vi "SDF Alarms.vi"(0 "Str Refnum":refnum<vi>, 5 "DigNum Refnum":refnum<vi>, 7 "High High":dbl, 9 "High":dbl, 11 "LC-test":dbl, 12 "LOW":dbl, 13 "LOW LOW":dbl, 14 "Reset":bool) -> (4 "String":string, 6 "Alarm":bool, 8 "Alarm Horn":bool, 10 "Warning Horn":bool, 15 "Warning":bool)   [LabVIEW 2013]
panel:
  out "Alarm Lolo":bool
  out "Alarm Hihi":bool
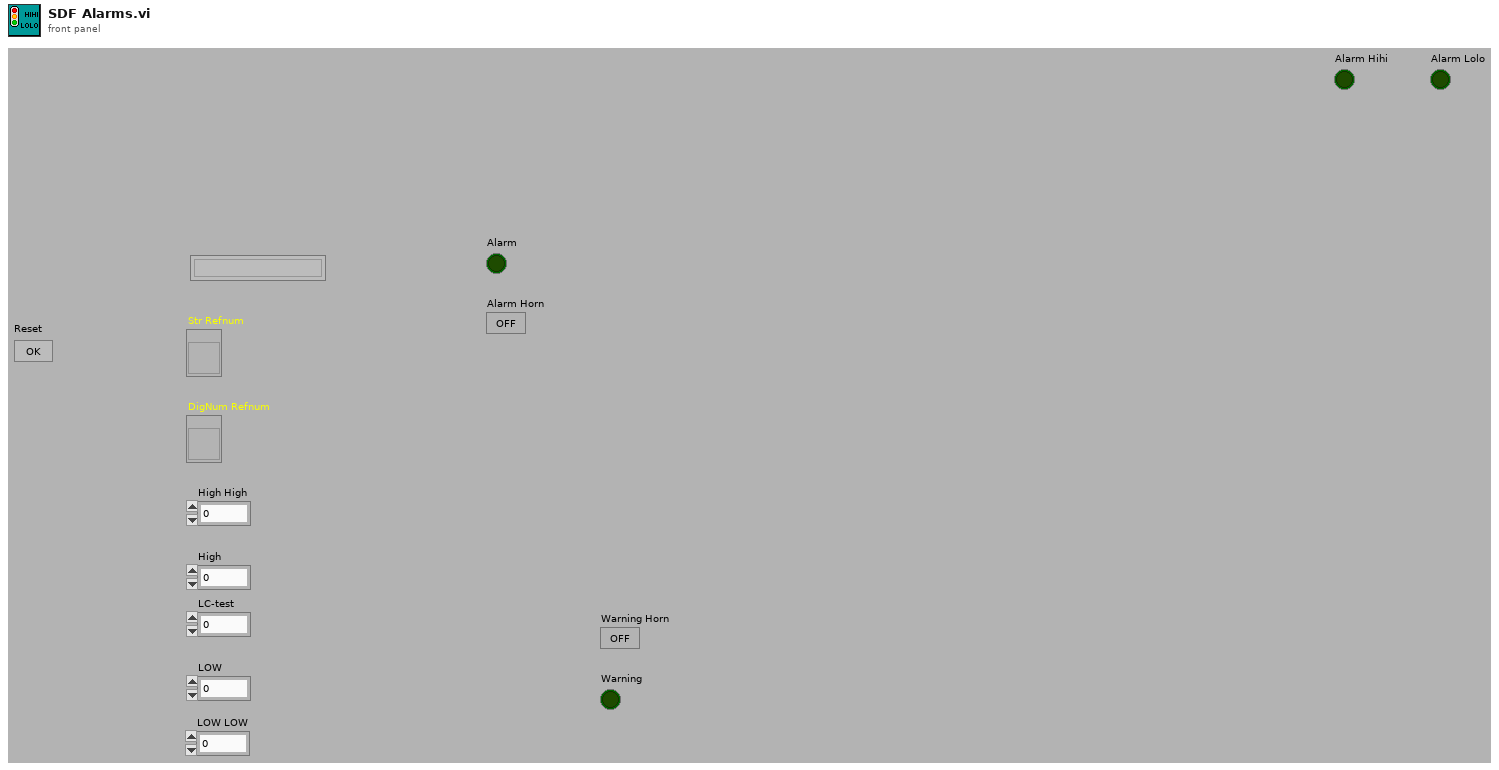
[diagram p1: front panel]
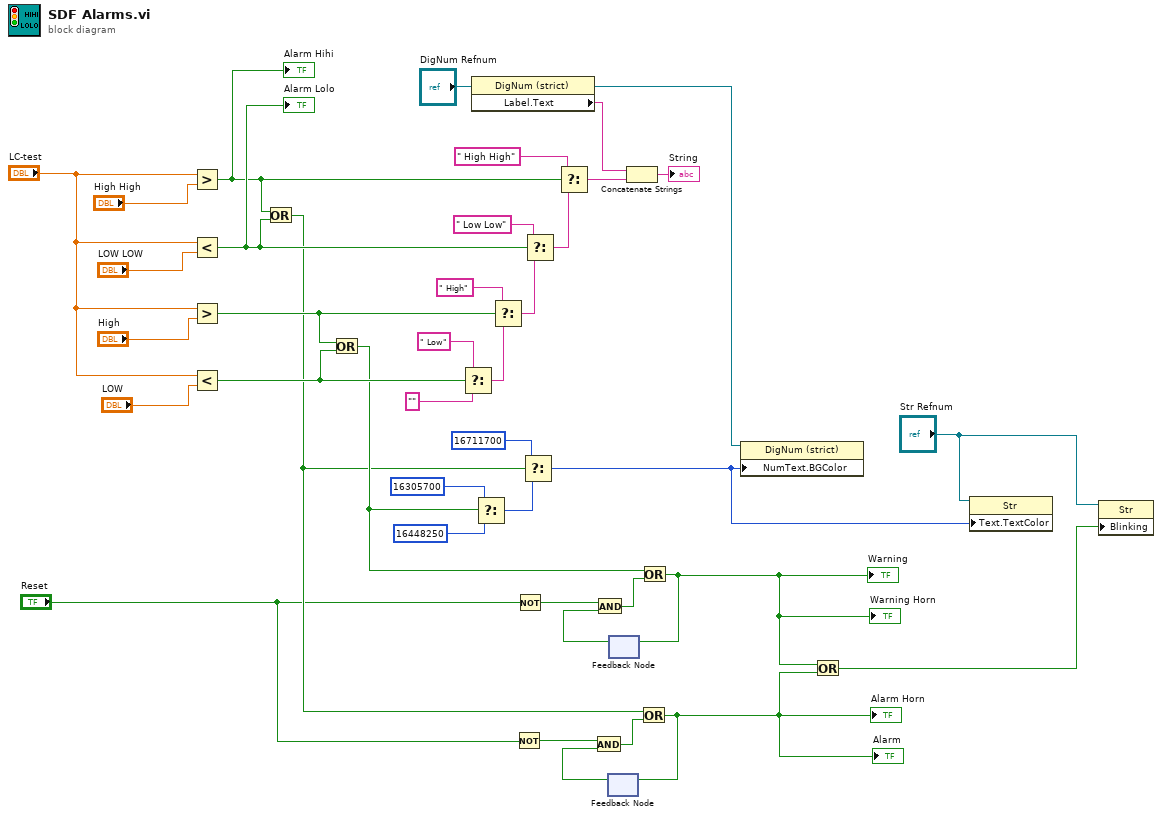
[diagram p0: block diagram]
diagram:
  n1 = Greater?(x="LC-test", y="High High") -> (0:w20:bool)
  "Alarm Hihi" <- w20
  n2 = Less?(x="LC-test", y="LOW LOW") -> (x < y?=w21:bool)
  "Alarm Lolo" <- w21
  n3 = Greater?(x="LC-test", y="High") -> (0:w28:bool)
  n4 = Less?(x="LC-test", y="LOW") -> (x < y?=w37:bool)
  n5 = Or(x=w20, y=w21) -> (x .or. y?=w9:bool)
  n6 = Or(x=w28, y=w37) -> (x .or. y?=w10:bool)
  n7 = Select(t=" Low", s=w37, f="") -> (s? t:f=w29:string)
  n8 = property on="Property Node" class="DigNum (strict)"(reference="DigNum Refnum") -> ("Label.Text"=w4:string)  [unwired: 1 in, 2 out]
  n9 = Select(t=16305700, s=w10, f=16448250) -> (s? t:f=w12:i32)
  n10 = Select(t=" High", s=w28, f=w29) -> (s? t:f=w30:string)
  n11 = Not(x="Reset") -> (.not. x?=w23:bool)
  n12 = Not(x="Reset") -> (.not. x?=w26:bool)
  n13 = Select(t=16711700, s=w9, f=w12) -> (s? t:f=w8:i32)
  n14 = Select(t=" Low Low", s=w21, f=w30) -> (s? t:f=w31:string)
  n15 = Select(t=" High High", s=w20, f=w31) -> (s? t:f=w5:string)
  n16 = feedback #1() -> (w24:bool)  [unwired: 1 in]
  n17 = And(x=w23, y=w24) -> (x .and. y?=w22:bool)
  n18 = feedback #2() -> (w27:bool)  [unwired: 1 in]
  n19 = And(x=w26, y=w27) -> (x .and. y?=w25:bool)
  n20 = Concatenate Strings(w4, w5) -> (→"String":string)
  n21 = Or(x=w9, y=w22) -> (x .or. y?=w1:bool)
  "Alarm" <- w1
  "Alarm Horn" <- w1
  n22 = feedback-in #1(w1) -> ()
  n23 = Or(x=w10, y=w25) -> (x .or. y?=w2:bool)
  "Warning" <- w2
  "Warning Horn" <- w2
  n24 = feedback-in #2(w2) -> ()
  n25 = property class="DigNum (strict)"(reference="DigNum Refnum", "NumText.BGColor"=w8) -> ()  [unwired: 1 in, 2 out]
  n26 = Or(x=w2, y=w1) -> (x .or. y?=w7:bool)
  n27 = property on="Property Node" class="Str"(reference="Str Refnum", "Text.TextColor"=w8) -> ()  [unwired: 1 in, 2 out]
  n28 = property on="Property Node" class="Str"(reference="Str Refnum", "Blinking"=w7) -> ()  [unwired: 1 in, 2 out]
